vi "HINCRBY.vi"(6 "integer value":i64, 8 "error in (no error)":errorcluster, 9 "field":string, 10 "key":string, 11 "Redis Client in":refnum<class "Redis Client.lvclass">) -> (0 "error out":errorcluster, 1 "new value":i64, 3 "Redis Client out":refnum<class "Redis Client.lvclass">)   [LabVIEW 2019, in "Redis Client for LabVIEW.lvlib" / "Redis Client.lvclass"]
uses:
  Redis Client.lvclass
  RESP3 for LabVIEW/RESP3/types/RESP3 data type attribute.vi
  RESP3 for LabVIEW/RESP3/high-level/RESP3 Get String.vi
  RESP3 for LabVIEW/RESP3/RESP3.lvlib
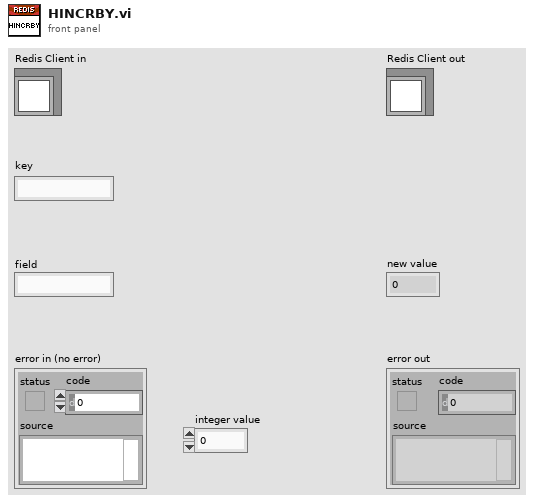
[diagram p1: front panel]
types:
  T1 = typedef "RESP3.lvlib/RESP3 Type.ctl" = enum8{"<0x00>", "<0x01>", "<0x02>", "<0x03>", "<0x04>", "<0x05>", "<0x06>", "<0x07>", "<0x08>", "<0x09>", "<0x0A>", "<0x0B>", "<0x0C>", "<0x0D>", "<0x0E>", "<0x0F>", "<0x10>", "<0x11>", "<0x12>", "<0x13>", "<0x14>", "<0x15>", "<0x16>", "<0x17>", "<0x18>", "<0x19>", "<0x1A>", "<0x1B>", "<0x1C>", "<0x1D>", "<0x1E>", "<0x1F>", "\" \"", "BLOB ERROR", "\"\"\"", "BOOLEAN", "BLOB", "MAP", "\"&\"", "\"'\"", "BIG NUMBER", "\")\"", "ARRAY", "STRING", "DOUBLE", "ERROR", "END", "\"/\"", "\"0\"", "\"1\"", "\"2\"", "\"3\"", "\"4\"", "\"5\"", "\"6\"", "\"7\"", "\"8\"", "\"9\"", "INTEGER", "STREAM", "\"<\"", "VERBATIM STRING", "PUSH", "\"?\"", "\"@\"", "\"A\"", "\"B\"", "\"C\"", "\"D\"", "\"E\"", "\"F\"", "\"G\"", "\"H\"", "\"I\"", "\"J\"", "\"K\"", "\"L\"", "\"M\"", "\"N\"", "\"O\"", "\"P\"", "\"Q\"", "\"R\"", "\"S\"", "\"T\"", "\"U\"", "\"V\"", "\"W\"", "\"X\"", "\"Y\"", "\"Z\"", "\"[\"", "\"\\\"", "\"]\"", "\"^\"", "NULL", "\"`\"", "\"a\"", "\"b\"", "\"c\"", "\"d\"", "\"e\"", "\"f\"", "\"g\"", "\"h\"", "\"i\"", "\"j\"", "\"k\"", "\"l\"", "\"m\"", "\"n\"", "\"o\"", "\"p\"", "\"q\"", "\"r\"", "\"s\"", "\"t\"", "\"u\"", "\"v\"", "\"w\"", "\"x\"", "\"y\"", "\"z\"", "\"{\"", "ATTRIBUTES", "\"}\"", "SET", "<0x7F>", "<0x80>", "<0x81>", "<0x82>", "<0x83>", "<0x84>", "<0x85>", "<0x86>", "<0x87>", "<0x88>", "<0x89>", "<0x8A>", "<0x8B>", "<0x8C>", "<0x8D>", "<0x8E>", "<0x8F>", "<0x90>", "<0x91>", "<0x92>", "<0x93>", "<0x94>", "<0x95>", "<0x96>", "<0x97>", "<0x98>", "<0x99>", "<0x9A>", "<0x9B>", "<0x9C>", "<0x9D>", "<0x9E>", "<0x9F>", "<0xA0>", "<0xA1>", "<0xA2>", "<0xA3>", "<0xA4>", "<0xA5>", "<0xA6>", "<0xA7>", "<0xA8>", "<0xA9>", "<0xAA>", "<0xAB>", "<0xAC>", "<0xAD>", "<0xAE>", "<0xAF>", "<0xB0>", "<0xB1>", "<0xB2>", "<0xB3>", "<0xB4>", "<0xB5>", "<0xB6>", "<0xB7>", "<0xB8>", "<0xB9>", "<0xBA>", "<0xBB>", "<0xBC>", "<0xBD>", "<0xBE>", "<0xBF>", "<0xC0>", "<0xC1>", "<0xC2>", "<0xC3>", "<0xC4>", "<0xC5>", "<0xC6>", "<0xC7>", "<0xC8>", "<0xC9>", "<0xCA>", "<0xCB>", "<0xCC>", "<0xCD>", "<0xCE>", "<0xCF>", "<0xD0>", "<0xD1>", "<0xD2>", "<0xD3>", "<0xD4>", "<0xD5>", "<0xD6>", "<0xD7>", "<0xD8>", "<0xD9>", "<0xDA>", "<0xDB>", "<0xDC>", "<0xDD>", "<0xDE>", "<0xDF>", "<0xE0>", "<0xE1>", "<0xE2>", "<0xE3>", "<0xE4>", "<0xE5>", "<0xE6>", "<0xE7>", "<0xE8>", "<0xE9>", "<0xEA>", "<0xEB>", "<0xEC>", "<0xED>", "<0xEE>", "<0xEF>", "<0xF0>", "<0xF1>", "<0xF2>", "<0xF3>", "<0xF4>", "<0xF5>", "<0xF6>", "<0xF7>", "<0xF8>", "<0xF9>", "<0xFA>", "<0xFB>", "<0xFC>", "<0xFD>", "<0xFE>"}
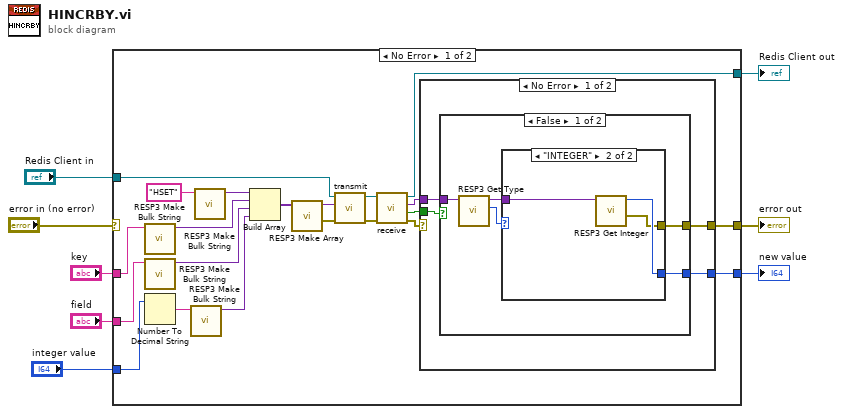
[diagram p0: block diagram]
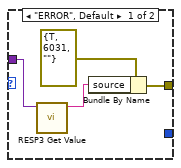
[diagram p2: hidden frame]
diagram:
  n1 = case shown="No Error" "error in (no error)" {
    selector: "error in (no error)" -> [_ w48]
    tunnel: [w21 w48] -> w7
    tunnel: "Redis Client in" -> [w29 w47]
    tunnel: [w26 w47] -> w5
    tunnel: "key" -> [w18 _]
    tunnel: "field" -> [w17 _]
    tunnel: [w20 _] -> w2
    tunnel: "integer value" -> [w10 _]
    frame No Error {
      n2 = call "RESP3 Make Bulk String.vi"("String"=w18) -> ("RESP3 Value out"=w15:variant)  [unwired: 9 in, 1 out]
      n3 = call "RESP3 Make Bulk String.vi"("String"=w17) -> ("RESP3 Value out"=w14:variant)  [unwired: 9 in, 1 out]
      n4 = Number To Decimal String(number=w10) -> (decimal integer string=w9:string)  [unwired: 1 in]
      n5 = call "RESP3 Make Bulk String.vi"("String"=w9) -> ("RESP3 Value out"=w11:variant)  [unwired: 9 in, 1 out]
      n6 = call "RESP3 Make Bulk String.vi"("String"="HSET" ("string in")) -> ("RESP3 Value out"=w16:variant)  [unwired: 9 in, 1 out]
      n7 = Build Array(w16, w15, w14, w11) -> (w28:variant[])
      n8 = call "RESP3 Make Array.vi"("RESP3 Values in"=w28) -> ("error out"=w13:errorcluster, "RESP3 Value out"=w12:variant)  [unwired: 9 in]
      n9 = call-dynamic "transmit.vi"("error in (no error)"=w13, "RESP3 Value"=w12, "Redis Client in"=w29) -> ("error out"=w25:errorcluster, "Redis Client out"=w27:refnum<class "Redis Client.lvclass">)  [unwired: 7 in]
      n10 = call-dynamic "receive.vi"("error in (no error)"=w25, "Redis Client in"=w27) -> ("error out"=w24:errorcluster, "timed out?"=w23:bool, "RESP3 Value"=w22:variant, "Redis Client out"=w26:refnum<class "Redis Client.lvclass">)  [unwired: 6 in]
      n11 = case shown="No Error" w24 {
        selector: w24 -> [_ w46]
        tunnel: [w33 _] -> w20
        tunnel: [w32 w46] -> w21
        tunnel: w22 -> [w30 _]
        tunnel: w23 -> [w31 _]
        frame No Error {
          n12 = case shown="False" w31 {
            tunnel: [w38 _] -> w33
            tunnel: [w37 _] -> w32
            tunnel: w30 -> [w36 _]
            frame False {
              n13 = call "RESP3 Get Type.vi"("RESP3 Value in"=w36) -> ("RESP3 Type"=w34:T1, "RESP3 Value out"=w35:variant)  [unwired: 7 in, 2 out]
              n14 = case shown="\"INTEGER\"" w34 {
                tunnel: [_ w45] -> w38
                tunnel: [w41 w44] -> w37
                tunnel: w35 -> [w40 w43]
                frame "ERROR", Default {
                  n15 = call-poly "RESP3 Get Value.vi"("RESP3 Value in"=w40) -> ("String out"=w39:string)  [unwired: 7 in, 3 out]
                  n16 = Bundle By Name(cluster=errorcluster {"status"=TRUE, "code"=6031, "source"=""} ("error constant"), "source"=w39) -> (w41:errorcluster)
                }
                frame "INTEGER" {
                  n17 = call "RESP3 Get Integer.vi"("RESP3 Value in"=w43) -> ("error out"=w44:errorcluster, "I64 out"=w45:i64)  [unwired: 8 in, 1 out]
                }
              }
            }
            frame True {
            }
          }
        }
        frame Error {
        }
      }
    }
    frame Error {
    }
  }
  "error out" <- w7
  "Redis Client out" <- w5
  "new value" <- w2
